vi "Save Settings.vi"(8 "error in (no error)":errorcluster, 11 "IMAQ Display in":refnum<class "HIJ IMAQdx Display.lvclass">) -> (0 "error out":errorcluster, 3 "IMAQ Display out":refnum<class "HIJ IMAQdx Display.lvclass">)   [LabVIEW 2020, in "HIJ IMAQdx Display.lvlib" / "HIJ IMAQdx Display.lvclass"]
uses:
  HIJ IMAQdx Display.lvclass
  C:/POLARIS Programme/POLARIS-AS-3-Cams/Submodules/HIJ Vision/Display Actors/HIJ Vision Display/HIJ Vision Display/HIJ Vision Display.lvclass
  HIJ Vision Display/HIJ Vision Display/Named ROI.ctl
  HIJ Vision Display/HIJ Vision Display/DisplaySettings.ctl
  HIJ Vision Display/HIJ Vision Display/HIJ Vision Display.lvclass/HIJ Vision Display.ctl
  HIJ IMAQdx Display.lvclass/HIJ IMAQdx Display.ctl
  HIJ Vision Display/HIJ Vision Display/Read Image Source Name.vi
  HIJ Vision Display/HIJ Vision Display/Read Display settings.vi
  HIJ Vision Display/HIJ Vision Display/Read Saved ROIs.vi
  HIJ Vision Display/HIJ Vision Display/Read ROI.vi
  HIJ Vision Display/HIJ Vision Display/Read Display ref.vi
  Utility/POLARIS Vision utility.lvlib
  HIJ Vision Display/HIJ Vision Display/HIJ Vision Display.lvclass
panel:
  in  "ROI":T1 {"Contours"."Type" items=["No Selection", "Point", "Line", "Rectangle", "Oval", "Polygon", "Freehand Region", "Annulus", "Unused2", "Unused3", "Broken Line", "Freehand Line", "Rotated Rectangle"]}
  in  "Display settings":T2
  in  "Image Center":cluster{"X":u32, "Y":u32}
  in  "Zoom":cluster{"X":i32, "Y":i32}
  in  "Saved ROIs":T3[](array[typedef])
  out "Image":T4(plugin-control)
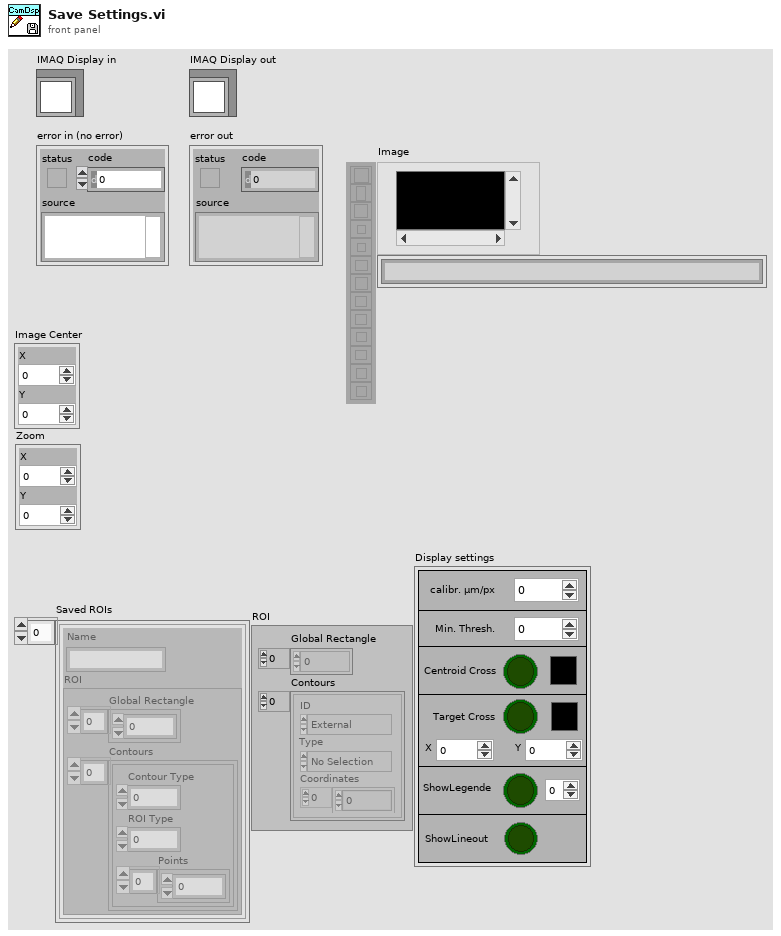
[diagram p1: front panel]
types:
  T1 = typedef "ROI Descriptor" = cluster{"Global Rectangle":i32[], "Contours":cluster{"ID":enum32{"External", "Internal"}, "Type":u32, "Coordinates":i32[]}[]}
  T2 = typedef "HIJ Vision Display.lvlib/HIJ Vision Display.lvclass/DisplaySettings.ctl" = cluster{"Min. Thresh.":sgl, "X":dbl, "Y":dbl, "ShowLineout":bool, "ScaleParts":i32, "ShowLegende":bool, "Target Cross":bool, "Centroid Cross":bool, "Target color":u32, "Centroid color":u32, "calibr. µm/px":sgl[unit]}
  T3 = typedef "HIJ Vision Display.lvlib/HIJ Vision Display.lvclass/Named ROI.ctl" = cluster{"ROI":cluster{"Global Rectangle":i32[], "Contours":cluster{"Contour Type":u32, "ROI Type":u32, "Points":i32[]}[]}, "Name":string}
  T4 = typedef "IMAQ Image.ctl" = refnum<image>
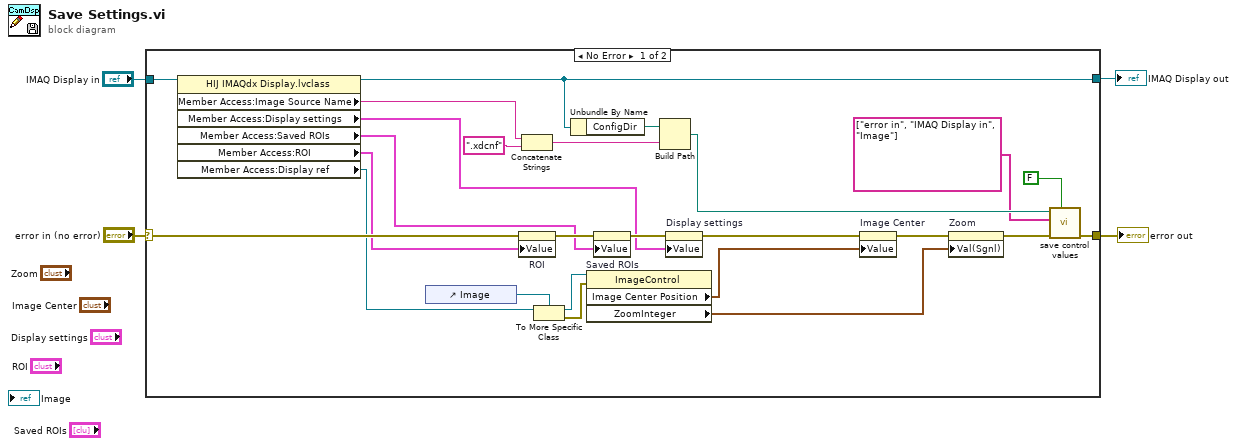
[diagram p0: block diagram]
diagram:
  n1 = case shown="No Error" "error in (no error)" {
    selector: "error in (no error)" -> [w27 w31]
    tunnel: [w26 w31] -> w1
    tunnel: [w25 w30] -> w3
    tunnel: "IMAQ Display in" -> [w28 w30]
    frame No Error {
      n2 = property class="HIJ IMAQdx Display.lvclass"(reference=w28) -> (reference out=w25:refnum<class "HIJ IMAQdx Display.lvclass">, "Member Access:Image Source Name"=w6:string, "Member Access:Display settings"=w5:T2, "Member Access:Saved ROIs"=w7:T3[], "Member Access:ROI"=w8:T1, "Member Access:Display ref"=w12:refnum<vi>)  [unwired: 1 in, 1 out]
      n3 = control-ref of="Image"() -> (w21:refnum<vi>)
      n4 = property on="ROI" class="Clust (strict)"(error in=w27, "Value"=w8) -> (error out=w11:errorcluster)  [unwired: 1 in, 1 out]
      n5 = Concatenate Strings(w6, ".xdcnf" ("string")) -> (w15:string)
      n6 = To More Specific Class(target class=w21, reference=w12) -> (specific class reference=w20:refnum<vi>, error out=w19:errorcluster)  [unwired: 1 in]
      n7 = Unbundle By Name(w25) -> ("ConfigDir"=w29:path)
      n8 = property class="ImageControl"(reference=w20, error in=w19) -> ("Image Center Position"=w22:cluster{"X":u32, "Y":u32}, "ZoomInteger"=w23:cluster{"X":i32, "Y":i32})  [unwired: 2 out]
      n9 = property on="Saved ROIs" class="Arr (strict)"(error in=w11, "Value"=w7) -> (error out=w10:errorcluster)  [unwired: 1 in, 1 out]
      n10 = Build Path(base path=w29, name or relative path=w15) -> (appended path=w18:path)
      n11 = property on="Display settings" class="Clust (strict)"(error in=w10, "Value"=w5) -> (error out=w9:errorcluster)  [unwired: 1 in, 1 out]
      n12 = property on="Image Center" class="Clust (strict)"(error in=w9, "Value"=w22) -> (error out=w14:errorcluster)  [unwired: 1 in, 1 out]
      n13 = property on="Zoom" class="Clust (strict)"(error in=w14, "Val(Sgnl)"=w23) -> (error out=w13:errorcluster)  [unwired: 1 in, 1 out]
      n14 = call "save control values.vi"("Append timestamp (true)"=FALSE, "error in"=w13, "Dont save"=string[] ["error in", "IMAQ Display in", "Image"], "Path"=w18) -> ("error out"=w26:errorcluster)  [unwired: 4 in, 1 out]
    }
    frame Error {
    }
  }
  "IMAQ Display out" <- w3
  "error out" <- w1
